vi "Write DWA.vi"(10 "Parameter Cluster":T1, 11 "Toggle 7.1 in":refnum<class "Toggle 7.1.lvclass">) -> (3 "Toggle 7.1 out":refnum<class "Toggle 7.1.lvclass">)   [LabVIEW 2020, in "Toggle 7.1.lvclass"]
uses:
  Toggle 7.1.lvclass
  Controls/Parameter Cluster.ctl
  Toggle 7.1.lvclass/Toggle 7.1.ctl
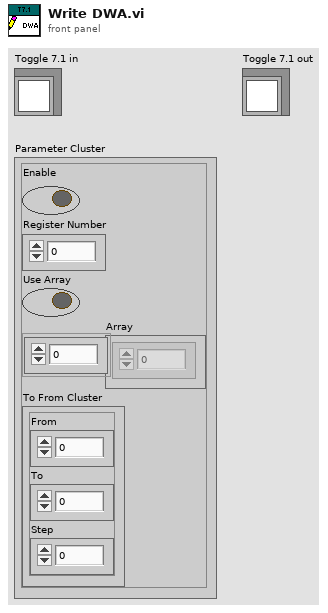
[diagram p1: front panel]
types:
  T1 = typedef "Toggle 7.1.lvclass/Parameter Cluster.ctl" = cluster{"Enable":bool, "Register Number":u32, "Use Array":bool, "Array":dbl[], "To From Cluster":cluster{"From":dbl, "To":dbl, "Step":dbl}}
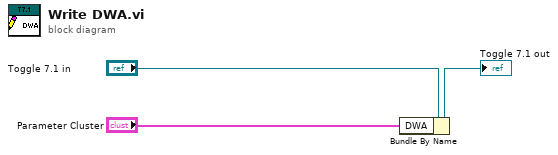
[diagram p0: block diagram]
diagram:
  n1 = Bundle By Name(cluster="Toggle 7.1 in", "DWA"="Parameter Cluster") -> (→"Toggle 7.1 out":refnum<class "Toggle 7.1.lvclass">)
